vi "ServerDemo.vi"() -> ()   [LabVIEW 2010]
uses:
  lib/Snap7.lvlib
panel:
  out "ServerStatus":i32(ring)=1 items=["Stop", "Run", "Error"]
  out "CpuStatus":i32(ring)=8 items=["Run"=8, "Stop"=4]
  out "ClientsCount":i32
  out "Log":string
  in  "stop":bool
  in  "Address":string="0.0.0.0"
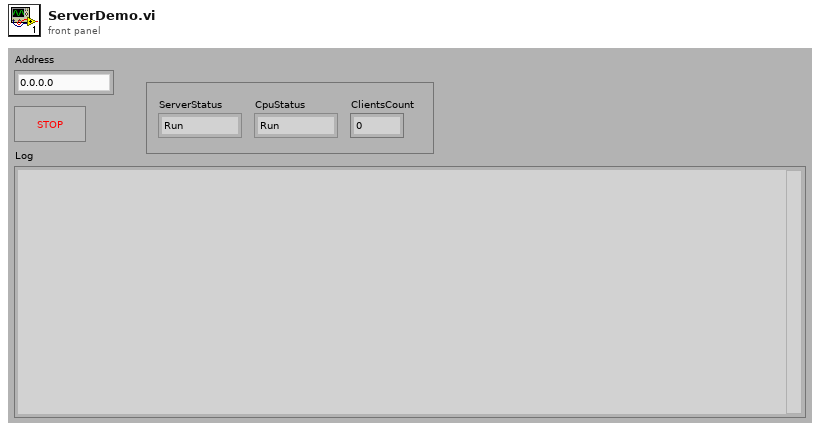
[diagram p1: front panel]
types:
  T1 = enum16{"big-endian, network order", "native, host order", "little-endian"}
  T2 = cluster{"evtTime":u32, "evtSender":i32, "evtCode":u32, "evtRetCode":u16, "evtParam1":u16, "evtParam2":u16, "evtParam3":u16, "evtParam4":u16}
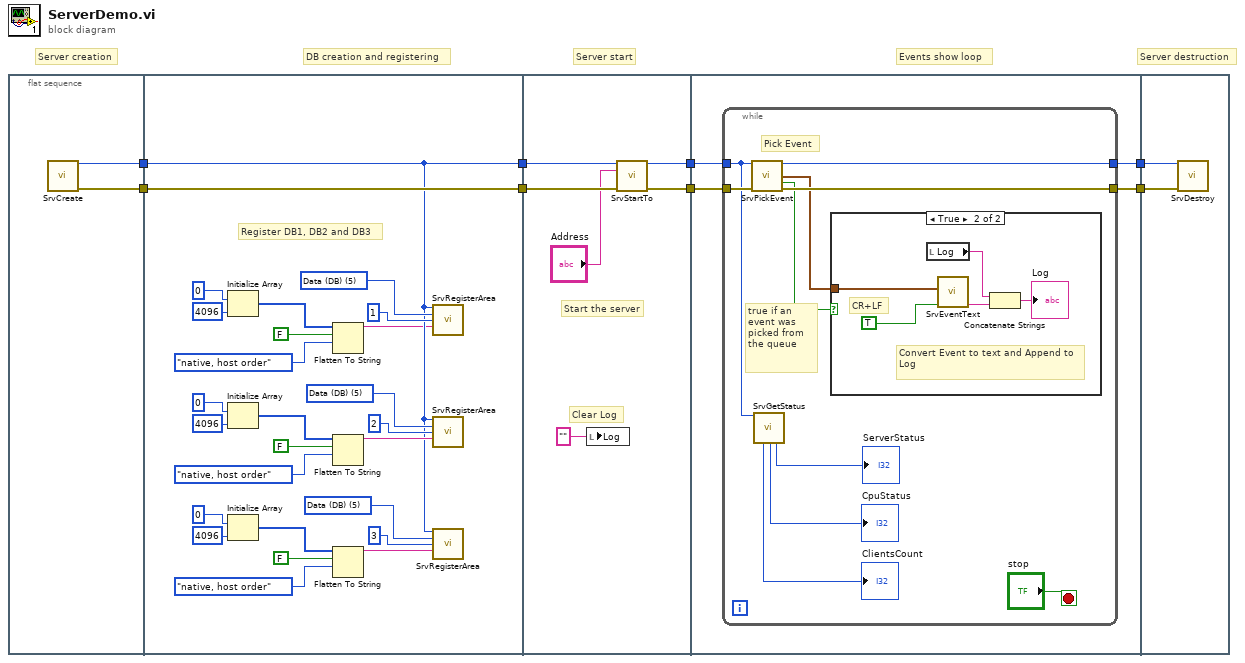
[diagram p0: block diagram]
diagram:
  # "Server destruction"
  # "Events show loop"
  # "Server start"
  # "DB creation and registering"
  # "Server creation"
  n1 = flat-sequence {
    tunnel: [w10] -> w7
    tunnel: [w9] -> w5
    tunnel: [w12] -> w8
    tunnel: w7 -> [w12]
    tunnel: [w36] -> w6
    tunnel: w5 -> [w36]
    tunnel: w8 -> [w42]
    tunnel: w6 -> [w41]
    tunnel: [w39] -> w3
    tunnel: [w38] -> w2
    tunnel: [w45] -> w4
    tunnel: w3 -> [w46]
    tunnel: w2 -> [w44]
    tunnel: [w43] -> w1
    tunnel: w4 -> [w63]
    tunnel: w1 -> [w62]
    frame #0 {
      n2 = call "SrvCreate.vi"() -> ("ref out"=w10:u64, "error out"=w9:errorcluster)  [unwired: 14 in]
    }
    frame #1 {
      w13 = 5 items=["Inputs (EB)", "Output (AB)", "Bit Memory (M)", "Counters (Z)", "Timers (T)", "Data (DB)"] ("AreaCode")
      w14 = 5 items=["Inputs (EB)", "Output (AB)", "Bit Memory (M)", "Counters (Z)", "Timers (T)", "Data (DB)"] ("AreaCode")
      w15 = 5 items=["Inputs (EB)", "Output (AB)", "Bit Memory (M)", "Counters (Z)", "Timers (T)", "Data (DB)"] ("AreaCode")
      # "Register DB1, DB2 and DB3"
      n3 = Initialize Array(u8 0, 4096) -> (w33:u8[])
      n4 = Initialize Array(u8 0, 4096) -> (w28:u8[])
      n5 = Initialize Array(u8 0, 4096) -> (w22:u8[])
      n6 = Flatten To String(anything=w33, prepend array or string size? (T)=FALSE, byte order (0:big-endian, network order)=T1."native, host order") -> (data string=w11:string)  [unwired: 1 in, 2 out]
      n7 = Flatten To String(anything=w28, prepend array or string size? (T)=FALSE, byte order (0:big-endian, network order)=T1."native, host order") -> (data string=w25:string)  [unwired: 1 in, 2 out]
      n8 = Flatten To String(anything=w22, prepend array or string size? (T)=FALSE, byte order (0:big-endian, network order)=T1."native, host order") -> (data string=w19:string)  [unwired: 1 in, 2 out]
      n9 = call "SrvRegisterArea.vi"("ref in"=w12, "AreaCode"=w15, "Index"=u16 1, "data in"=w11) -> ()  [unwired: 8 in, 4 out]
      n10 = call "SrvRegisterArea.vi"("ref in"=w12, "AreaCode"=w14, "Index"=u16 2, "data in"=w25) -> ()  [unwired: 8 in, 4 out]
      n11 = call "SrvRegisterArea.vi"("ref in"=w12, "AreaCode"=w13, "Index"=u16 3, "data in"=w19) -> ()  [unwired: 8 in, 4 out]
    }
    frame #2 {
      # "Start the server"
      # "Clear Log"
      n12 = local write "Log"("" ("Log")) -> ()
      n13 = call "SrvStartTo.vi"("ref in"=w42, "Address"="Address", "error in (no error)"=w41) -> ("ref out"=w39:u64, "error out"=w38:errorcluster)  [unwired: 10 in, 1 out]
    }
    frame #3 {
      n14 = while {
        tunnel: w46 -> [w50]
        tunnel: [w55] -> w45
        tunnel: w44 -> [w54]
        tunnel: [w53] -> w43
        stop <- "stop" stop-if-true
        # "Pick Event"
        # "true if an event was picked from the queue"
        n15 = call "SrvPickEvent.vi"("ref in"=w50, "error in (no error)"=w54) -> ("ref out"=w55:u64, "Event"=w52:T2, "EventReady"=w51:bool, "error out"=w53:errorcluster)  [unwired: 9 in, 1 out]
        n16 = call "SrvGetStatus.vi"("ref in"=w50) -> ("ClientsCount"=→"ClientsCount":i32, "CpuStatus"=→"CpuStatus":i32, "ServerStatus"=→"ServerStatus":i32)  [unwired: 9 in, 3 out]
        n17 = case shown="True" w51 {
          tunnel: w52 -> [_ w61]
          frame False {
            # "No event ready : nothing to do"
          }
          frame True {
            # "Convert Event to text and Append to Log"
            # "CR+LF"
            n18 = local read "Log"() -> (w58:string)
            n19 = call "SrvEventText.vi"("CR_LF"=TRUE, "var_Event"=w61) -> ("EventText"=w57:string)  [unwired: 7 in, 1 out]
            n20 = Concatenate Strings(w58, w57) -> (→"Log":string)
          }
        }
      }
    }
    frame #4 {
      n21 = call "SrvDestroy.vi"("ref in"=w63, "error in (no error)"=w62) -> ()  [unwired: 13 in, 1 out]
    }
  }
